vi "Init Device.vi"(7 "Layout Ref":refnum<vi>, 8 "error in (no error)":errorcluster, 10 "Chan# Array":i32[](array[numeric]), 11 "DMD in":refnum<class "DMD.lvclass">) -> (0 "error out":errorcluster, 3 "DMD out":refnum<class "DMD.lvclass">)   [LabVIEW 2013, in "DMD.lvclass"]
doc: "Initialize the correct columns and their default appearance.\nUse the front panel to change default appearance of the device in the Add/Manage devices.\n\nOpen a specific device implementation for details."
uses:
  DMD.lvclass
  ColumnVIs/SingleValCol/SingleValCol.lvclass
  ColumnVIs/SingleValMenuCol/SingleValMenuCol.lvclass
  TypeDefs/ColumnAppearCluster.ctl
  ColumnVIs/Column/Column.lvclass
panel:
  in  "Program Mode Appearance":T1={"Column Name"="Program Mode", "Width"=30, "Bkgd"=[16448250], "Text"=[0]}
  in  "MenuItemList 2":string[](array[string])=["Always Upload", "Upload Changes Only"]
  in  "Pattern Name Appearance":T1={"Column Name"="Pattern Name", "Width"=30, "Bkgd"=[16448250], "Text"=[0]}
  in  "Imgs in Pattern Appearance":T1={"Column Name"="Num Images", "Width"=30, "Bkgd"=[16448250], "Text"=[0]}
  in  "Display Mode Appearance":T1={"Column Name"="Disp Mode", "Width"=30, "Bkgd"=[16448250], "Text"=[0]}
  in  "MenuItemList":string[](array[string])=["Static Image", "Pattern Sequence"]
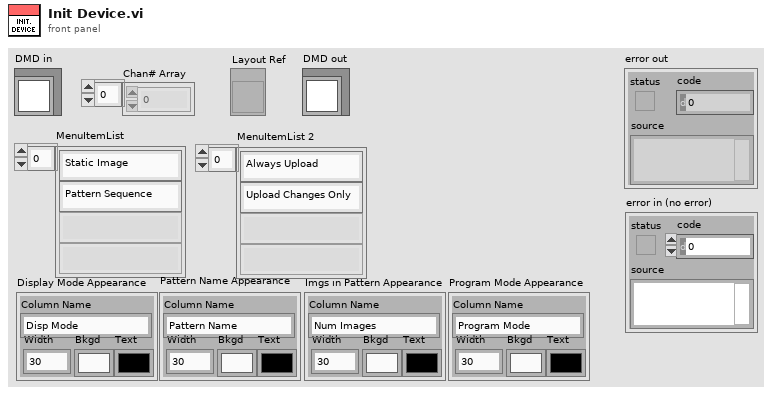
[diagram p1: front panel]
types:
  T1 = typedef "ColumnAppearCluster.ctl" = cluster{"Column Name":string, "Width":u32, "Bkgd":u32[], "Text":u32[]}
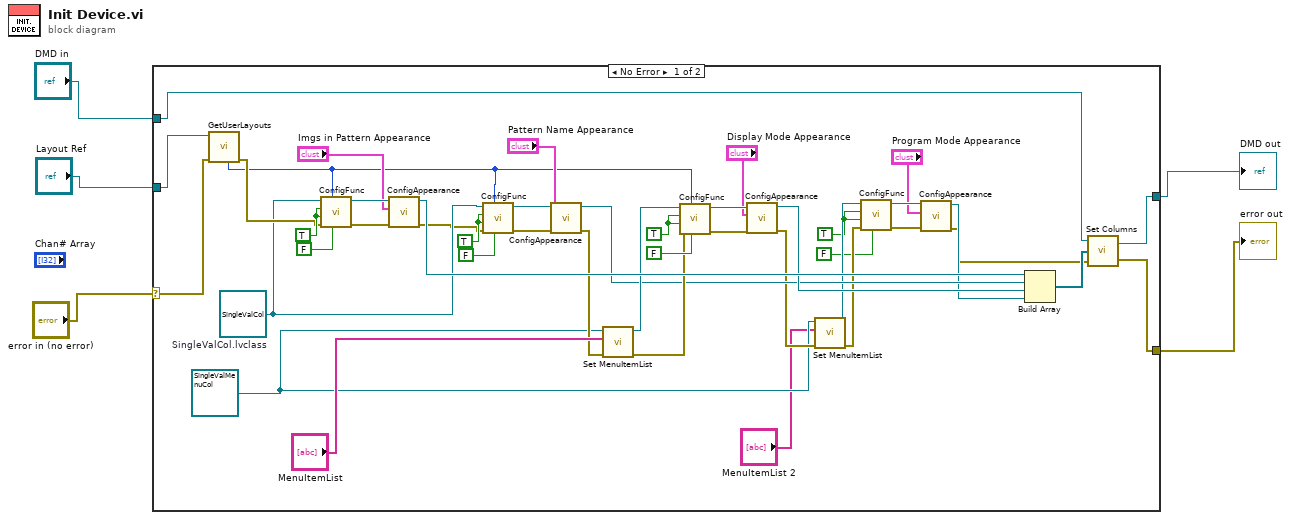
[diagram p0: block diagram]
diagram:
  n1 = case shown="No Error" "error in (no error)" {
    selector: "error in (no error)" -> [w48 w50]
    tunnel: "DMD in" -> [w38 w51]
    tunnel: [w37 w51] -> w2
    tunnel: [w33 w50] -> w3
    tunnel: "Layout Ref" -> [w49 _]
    frame No Error {
      w7 = TRUE ("Disableable? (True)")
      w26 = TRUE ("Disableable? (True)")
      w10 = refnum<class "SingleValMenuCol.lvclass"> refnum ("SingleValMenuCol.lvclass")
      w44 = TRUE ("Disableable? (True)")
      w46 = TRUE ("Disableable? (True)")
      w23 = refnum<class "SingleValCol.lvclass"> refnum  # SingleValCol.lvclass
      n2 = call "GetUserLayouts.vi"("error in (no error)"=w48, "Layout Ring Refnum"=w49) -> ("error out"=w36:errorcluster, "Num User Layouts"=w21:i32)  [unwired: 5 in, 3 out]
      n3 = call "ConfigFunc.vi"("isRampable? (True"=FALSE, "Num Layouts (ignored)"=w21, "error in (no error)"=w36, "isVariable? (True)"=w46, "Disableable? (True)"=w46, "Column in"=w23) -> ("error out"=w35:errorcluster, "Column out"=w47:refnum<class "SingleValCol.lvclass">)  [unwired: 4 in]
      n4 = call "ConfigAppearance.vi"("error in (no error)"=w35, "Column Appearance"="Imgs in Pattern Appearance", "Column in"=w47) -> ("error out"=w20:errorcluster, "Column out"=w41:refnum<class "SingleValCol.lvclass">)  [unwired: 7 in]
      n5 = call "ConfigFunc.vi"("isRampable? (True"=FALSE, "Num Layouts (ignored)"=w21, "error in (no error)"=w20, "isVariable? (True)"=w26, "Disableable? (True)"=w26, "Column in"=w23) -> ("error out"=w25:errorcluster, "Column out"=w27:refnum<class "SingleValCol.lvclass">)  [unwired: 4 in]
      n6 = call "ConfigAppearance.vi"("error in (no error)"=w25, "Column Appearance"="Pattern Name Appearance", "Column in"=w27) -> ("error out"=w19:errorcluster, "Column out"=w18:refnum<class "SingleValCol.lvclass">)  [unwired: 7 in]
      n7 = call-dynamic "Set MenuItemList.vi"("error in (no error)"=w19, "MenuItemList"="MenuItemList", "MenuCol in"=w10) -> ("error out"=w28:errorcluster, "MenuCol out"=w30:refnum<class "SingleValMenuCol.lvclass">)  [unwired: 7 in]
      n8 = call "ConfigFunc.vi"("isRampable? (True"=FALSE, "Num Layouts (ignored)"=w21, "error in (no error)"=w28, "isVariable? (True)"=w44, "Disableable? (True)"=w44, "Column in"=w30) -> ("error out"=w34:errorcluster, "Column out"=w45:refnum<class "SingleValMenuCol.lvclass">)  [unwired: 4 in]
      n9 = call "ConfigAppearance.vi"("error in (no error)"=w34, "Column Appearance"="Display Mode Appearance", "Column in"=w45) -> ("error out"=w12:errorcluster, "Column out"=w40:refnum<class "SingleValMenuCol.lvclass">)  [unwired: 7 in]
      n10 = call-dynamic "Set MenuItemList.vi"("error in (no error)"=w12, "MenuItemList"="MenuItemList 2", "MenuCol in"=w10) -> ("error out"=w11:errorcluster, "MenuCol out"=w8:refnum<class "SingleValMenuCol.lvclass">)  [unwired: 7 in]
      n11 = call "ConfigFunc.vi"("isRampable? (True"=FALSE, "error in (no error)"=w11, "isVariable? (True)"=w7, "Disableable? (True)"=w7, "Column in"=w8) -> ("error out"=w17:errorcluster, "Column out"=w16:refnum<class "SingleValMenuCol.lvclass">)  [unwired: 5 in]
      n12 = call "ConfigAppearance.vi"("error in (no error)"=w17, "Column Appearance"="Program Mode Appearance", "Column in"=w16) -> ("error out"=w13:errorcluster, "Column out"=w14:refnum<class "SingleValMenuCol.lvclass">)  [unwired: 7 in]
      n13 = Build Array(w41, w18, w40, w14) -> (w39:refnum<class "Column.lvclass">[])
      n14 = call-dynamic "Set Columns.vi"("error in (no error)"=w13, "Columns"=w39, "Device in"=w38) -> ("error out"=w33:errorcluster, "Device out"=w37:refnum<class "DMD.lvclass">)  [unwired: 1 in]
    }
    frame Error {
    }
  }
  "error out" <- w3
  "DMD out" <- w2
